vi "Interpolate.vi"(10 "X":sgl[](array[numeric]), 11 "Points interpolation":u32) -> (3 "Array":sgl[](array[numeric]))   [LabVIEW 2013]
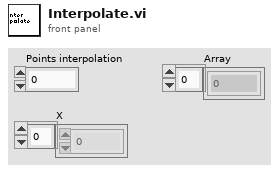
[diagram p1: front panel]
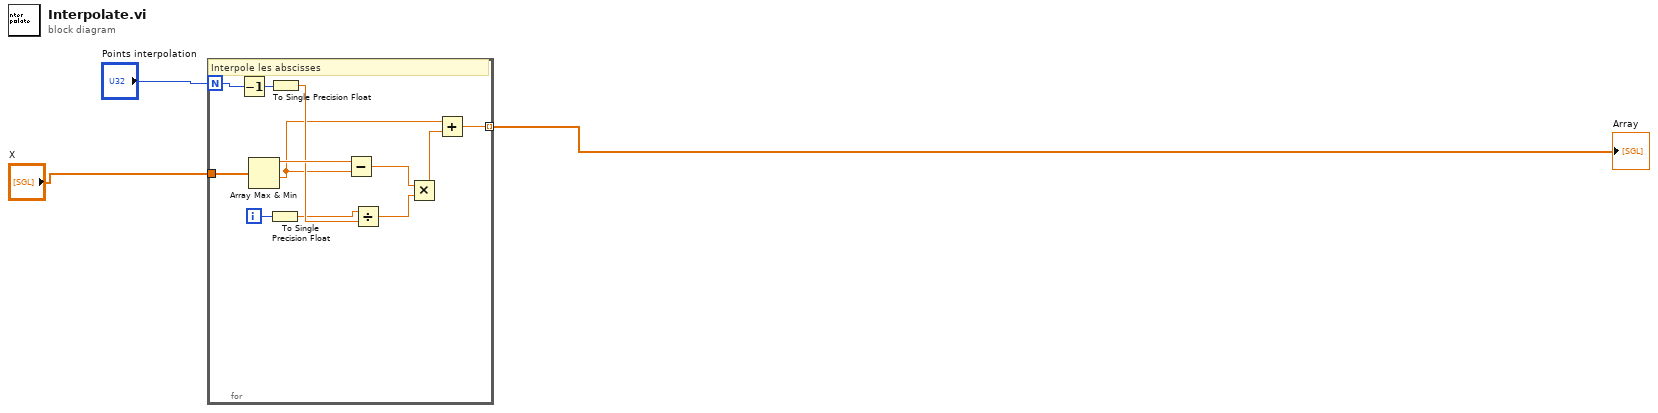
[diagram p0: block diagram]
diagram:
  n1 = for {
    N: "Points interpolation" -> [w15]
    tunnel: "X" -> [w14]
    tunnel: [w4] -> w3 mode=indexing
    i -> [w8]
    # "Interpole les abscisses"
    n2 = Decrement(x=w15) -> (x-1=w10:i32)
    n3 = Array Max & Min(array=w14) -> (max value=w11:sgl, min value=w5:sgl)  [unwired: 2 out]
    n4 = To Single Precision Float(number=w8) -> (single precision float=w7:sgl)
    n5 = To Single Precision Float(number=w10) -> (single precision float=w9:sgl)
    n6 = Subtract(x=w11, y=w5) -> (x-y=w13:sgl)
    n7 = Divide(x=w7, y=w9) -> (x/y=w12:sgl)
    n8 = Multiply(x=w13, y=w12) -> (x*y=w6:sgl)
    n9 = Add(x=w5, y=w6) -> (x+y=w4:sgl)
  }
  "Array" <- w3
